vi "Paskevits_Vladislav_2.vi"() -> ()   [LabVIEW 2018]
doc: "This Vi analyse temperature from the first VI, and also has to stop them."
uses:
  Paskevits_Vladislav_gbl1.vi
  Paskevits_Vladislav_gbl.vi
panel:
  in  "stop":bool
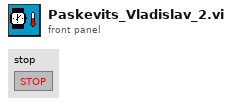
[diagram p1: front panel]
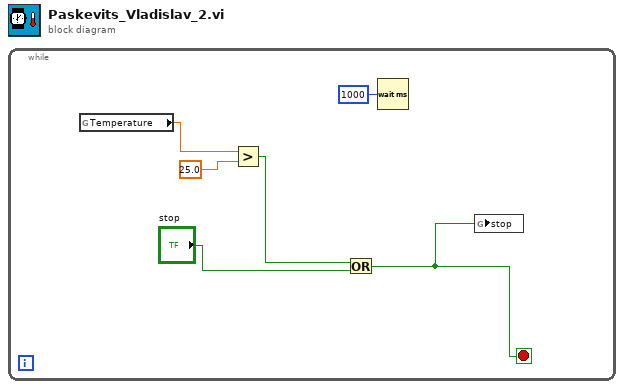
[diagram p0: block diagram]
diagram:
  n1 = while {
    stop <- w1 stop-if-true
    n2 = global read "Paskevits_Vladislav_gbl1.vi" "Temperature"() -> (w3:dbl)
    n3 = Greater?(x=w3, y=25.0) -> (0:w4:bool)
    n4 = Or(x=w4, y="stop") -> (x .or. y?=w1:bool)
    n5 = Wait (ms)(milliseconds to wait=u32 1000) -> ()  [unwired: 1 out]
    n6 = global write "Paskevits_Vladislav_gbl.vi" "stop"(w1) -> ()
  }
